vi "02-QNET_MECHKIT_Pressure_Sensor.vi"() -> ()   [LabVIEW 2012]
doc: "This VI is to be used with the NI-ELVIS and the QNET-Mechatronic Sensors I module. The objective is to calibrate the pressure sensor."
uses:
  <vilib>/Simulation/Scripting/Companion Diagram/SimConfigNode/SimParams.ctl
  <vilib>/Simulation/Scripting/Companion Diagram/SimConfigNode/_simSolvers.ctl
  <vilib>/Simulation/Implementation/Shared/SIMSCR Execution Mode.ctl
  <vilib>/Simulation/Param Hierarchy/Typedefs/SIMPH Param Control Actions.ctl
  <vilib>/Simulation/Implementation/Shared/NILVSim_ParamChanged.vi
  <vilib>/Simulation/SignalDisplay/Implementation/NILVSim Time Waveform.llb/SIM Time Waveform (scalar).vi
  <vilib>/Simulation/Utility/Implementation/SIM Halt.vi
  <vilib>/Simulation/Implementation/Shared/NILVSim_Manager.vi
  <vilib>/Simulation/Implementation/Shared/NILVSim_FinalizeModel.vi
  <vilib>/Simulation/Implementation/Shared/SIM Unbundle Sim Info.vi
  <vilib>/Utility/error.llb/Clear Errors.vi
  <vilib>/Simulation/Implementation/Shared/NILVSim_GetModelError.vi
  <vilib>/Simulation/Implementation/Shared/SIM Bundle Sim Info.vi
  <vilib>/Simulation/Implementation/Shared/SIMSH Read Queue.vi
  <vilib>/Simulation/Implementation/Shared/NILVSim_Initialize.vi
  <vilib>/Analysis/6fits.llb/General Polynomial Fit.vi
  <vilib>/DAQmx/read.llb/DAQmx Read.vi
  <vilib>/DAQmx/read.llb/DAQmx Read (Analog DBL 1Chan 1Samp).vi
  <vilib>/Simulation/Utility/Implementation/NILVSim Get Time and IsAcceptedStep.vi
  <vilib>/Simulation/Scripting/Companion Diagram/SimConfigNode/SimDog.xnode
  <vilib>/Simulation/Implementation/XNodeFramework/SimXNode/SimX.xnode
  <vilib>/Analysis/NI_AALPro.lvlib
  <vilib>/Simulation/Implementation/Shared/NI_SIM_Implementation.lvlib
panel:
  in  "Sampling Rate (Hz)":dbl=100.0 min=0.0 max=1000.0 step=25.0 format="%.1f"
  in  "Device":tag="Dev1"
  in  "Tab Control":enum32{"Collect Data", "Calibrate Sensor"}(tab)
  out "Presssure Sensor (V)":waveform(dbl)(graph)
  in  "Plunger Position (ml)":dbl[](array[numeric])=[1.0, 0.8, 0.6, 0.4, 0.2, 0.0]
  in  "Sensor Measurement (V)":dbl[](array[numeric])
  out "Sensor Readings":T1(graph)
  out "Coefficients: y = a*x^2 + b*x + c":dbl[](array[numeric]) format="%0.2f"
  out "Pressure (ml)":dbl(slide)
  in  "c (ml)":dbl
  in  "a (ml/V^2)":dbl
  out "Pressure Sensor (ml)":waveform(dbl)(graph)
  in  "b (ml/V)":dbl
  in  "stop":bool
  # "QNET-MECHKIT Pressure Sensor"
  # "NOTE 1: Place J9 jumper on \"Pressure\" setting.\nNOTE 2: Completely remove the plunger from the tube and re-insert it. This will\nensure the chamber is pressurized enough."
  # "1) Move the plunger to 1 ml.\n2) Enter measured sensor values in \"Sensor Measurement (V)\" array.\n3) Repeat for 0.8, 0.6, 0.4, 0.2, 0 ml."
  # "Polynomial curve fitting results:"
  # "c"
  # "b"
  # "a"
  # "Enter polynomial coefficients to measure correct position of the plunger\n(e.g. display below should read 0.5 ml when plunger at placed at 0.5 ml)."
  # "y = a*x^2 + b*x + c\nwhere\nx is the sensor voltage \ny is the output in millilitres."
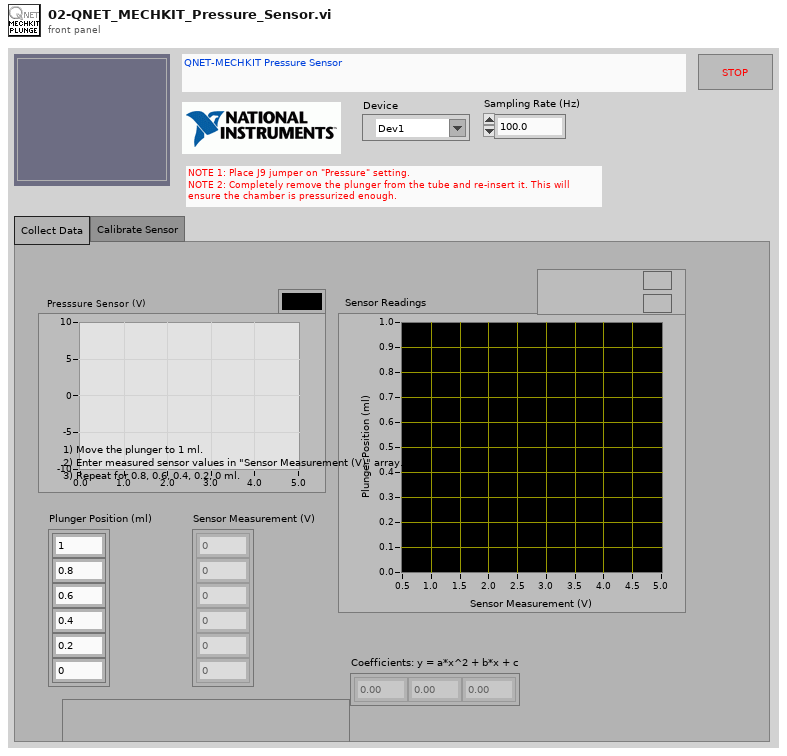
[diagram p1: front panel]
types:
  T1 = cluster{"Sensor Measurement (V)":dbl[], "Best Linear Fit":dbl[]}[]
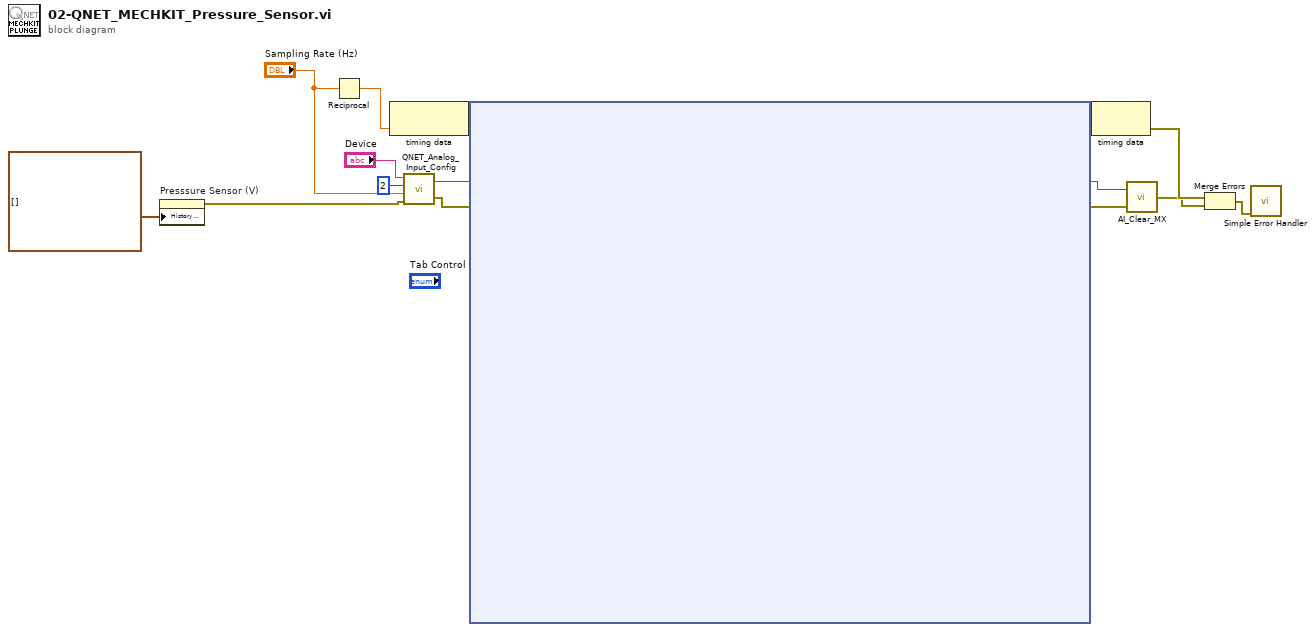
[diagram p0: block diagram]
diagram:
  n1 = property on="Presssure Sensor (V)" class="WFChart (strict)"("History Data"=waveform(dbl)[] []) -> (error out=w2:errorcluster)  [unwired: 2 in, 1 out]
  n2 = Reciprocal(x="Sampling Rate (Hz)") -> (1/x=w6:dbl)
  n3 = node-c288(w6) -> (w14:variant)
  n4 = call "QNET_Analog_Input_Config.vi"("error in"=w2, "sampling rate (Hz)"="Sampling Rate (Hz)", "analog input channel"=u32 2, "dev"="Device") -> ("error out"=w11:errorcluster, "task out"=w10:refnum<k21>)
  n5 = node-c254 ("Simulation Loop")(w14, w11, w10) -> (w13:variant, w9:refnum<k21>, w8:errorcluster)
  n6 = node-c288(w13) -> (w5:errorcluster)
  n7 = call "AI_Clear_MX.vi"("Error in"=w8, "Task in"=w9) -> ("Error out"=w4:errorcluster)
  n8 = Merge Errors(w5, w4) -> (w3:errorcluster)
  n9 = call <vilib>:"Simple Error Handler.vi"("error in (no error)"=w3) -> ()  [unwired: 1 in, 8 out]
